vi "Multiple Variable Names Dlg.vi"(10 "Variable Names in":string) -> (2 "Variable Names out":string, 3 "CONFIRM out":bool)   [LabVIEW 2015, in "Project.lvclass"]
uses:
  Project.lvclass
panel:
  in  "Variable Names":string
  in  "CANCEL":bool
  in  "CONFIRM":bool
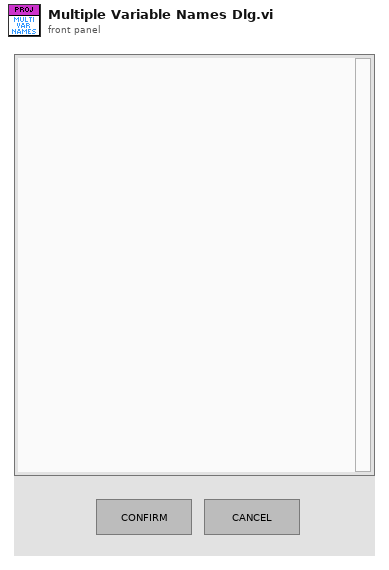
[diagram p1: front panel]
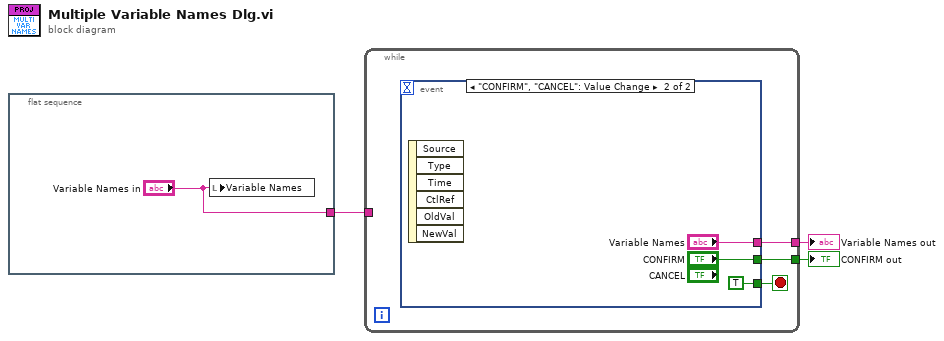
[diagram p0: block diagram]
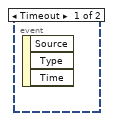
[diagram p2: hidden frame]
diagram:
  n1 = flat-sequence {
    tunnel: ["Variable Names in"] -> w1
    frame #0 {
      n2 = local write "Variable Names"("Variable Names in") -> ()
    }
  }
  n3 = while {
    tunnel: [w7] -> w3
    tunnel: [w5] -> w2
    tunnel: w1 -> [_]
    stop <- w6 stop-if-true
    n4 = event shown="[1] \"CONFIRM\", \"CANCEL\": Value Change" {
      selector: _ -> [_ _]
      dyn-events: _ -> [_ _]
      timeout: _ -> [_ _]
      tunnel: [_ "CONFIRM"] -> w7
      tunnel: [_ TRUE] -> w6
      tunnel: [_ "Variable Names"] -> w5
      event Timeout {
        n5 = event-data() -> ()  [unwired: 1 in, 3 out]
      }
      event "CONFIRM", "CANCEL": Value Change {
        n6 = event-data() -> ()  [unwired: 1 in, 6 out]
      }
    }
  }
  "CONFIRM out" <- w3
  "Variable Names out" <- w2
